vi "subPulseShapeandScale.vi"(0 "Symbol Stream":cdb[][](array[numeric]), 5 "pulse shaping filter coefficients":dbl[](array[numeric]) format="%.2f", 9 "samples per symbol (16)":i32=16, 11 "error in (no error)":errorcluster) -> (4 "Transmit Packets":cdb[][](array[numeric]), 15 "error out":errorcluster)   [LabVIEW 2011]
uses:
  <vilib>/addons/Modulation/Digital/General/MT Apply Pulse Shaping Filter (Generic).vi
  <vilib>/addons/Modulation/niDMT.lvlib
panel:
  in  "symbol rate (Hz)":dbl=1.0
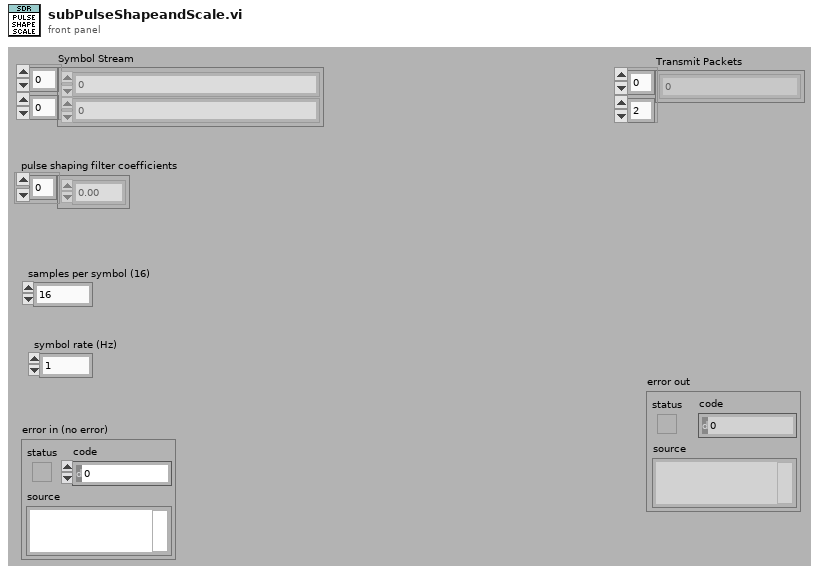
[diagram p1: front panel]
types:
  T1 = typedef "niAMT.lvlib/Complex Data Waveform.ctl" = cluster{"t0":dbl, "dt":dbl, "Y":cdb[]}
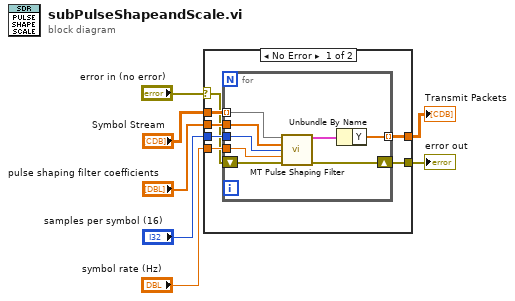
[diagram p0: block diagram]
diagram:
  n1 = case shown="No Error" "error in (no error)" {
    selector: "error in (no error)" -> [w8 w23]
    tunnel: [w12 w23] -> w6
    tunnel: "Symbol Stream" -> [w13 _]
    tunnel: "samples per symbol (16)" -> [w9 _]
    tunnel: [w14 _] -> w2
    tunnel: "pulse shaping filter coefficients" -> [w11 _]
    tunnel: "symbol rate (Hz)" -> [w10 _]
    frame No Error {
      n2 = for {
        tunnel: w13 -> [w21] mode=indexing
        shift-right: [w19] -> w12
        shift-left: w8 -> [w20]
        tunnel: [w22] -> w14 mode=indexing
        tunnel: w11 -> [w17]
        tunnel: w10 -> [w16]
        tunnel: w9 -> [w15]
        n3 = call-poly <vilib>:"MT Pulse Shaping Filter.vi"("symbols"=w21, "pulse shaping filter coefficients"=w17, "samples per symbol (16)"=w15, "symbol rate (Hz)"=w16, "error in (no error)"=w20) -> ("output complex waveform"=w18:T1, "error out"=w19:errorcluster)  [unwired: 9 in]
        n4 = Unbundle By Name(w18) -> ("Y"=w22:cdb[])
      }
    }
    frame Error {
    }
  }
  "error out" <- w6
  "Transmit Packets" <- w2
